vi "DriveTrainBoost (X) (Y).vi"(9 "Boost on":bool, 10 "axis 2 (y) in":dbl, 11 "axis 1 (x) in":dbl) -> (2 "axis 2 (y) out":dbl, 3 "axis 1 (x) out":dbl)   [LabVIEW 2012]
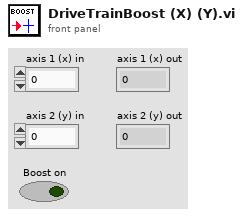
[diagram p1: front panel]
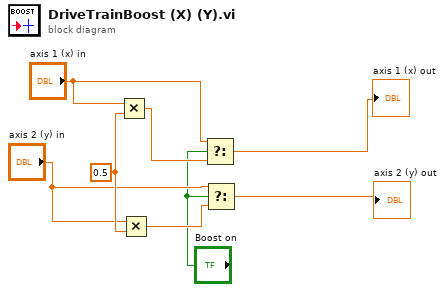
[diagram p0: block diagram]
diagram:
  w6 = 0.5 ("y")
  n1 = Multiply(x="axis 1 (x) in", y=w6) -> (x*y=w2:dbl)
  n2 = Multiply(x="axis 2 (y) in", y=w6) -> (x*y=w4:dbl)
  n3 = Select(t="axis 1 (x) in", s="Boost on", f=w2) -> (s? t:f=→"axis 1 (x) out":dbl)
  n4 = Select(t="axis 2 (y) in", s="Boost on", f=w4) -> (s? t:f=→"axis 2 (y) out":dbl)
